vi "Format Memory Cell to String.vi"(8 "error in (no error)":errorcluster, 10 "Format String":string, 11 "Memory Cell":T1) -> (0 "error out":errorcluster, 3 "output string":string)   [LabVIEW 2024]
uses:
  gScript Interpreter/Type Definitions/Memory Cell.ctl
  gScript Interpreter/Type Definitions/Memory Cell Type Enum.ctl
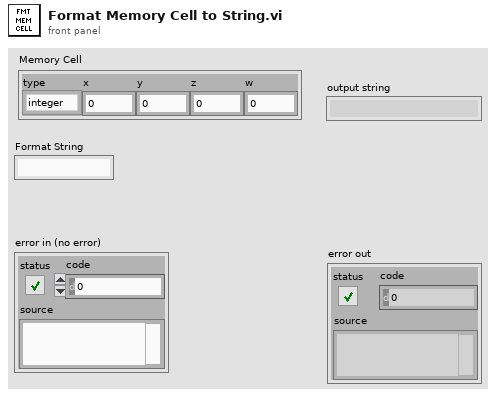
[diagram p1: front panel]
types:
  T1 = typedef "Memory Cell.ctl" = cluster{"type":T2, "x":dbl, "y":dbl, "z":dbl, "w":dbl}
  T2 = typedef "Memory Cell Type Enum.ctl" = enum16{"integer", "float", "vector", "rotation"}
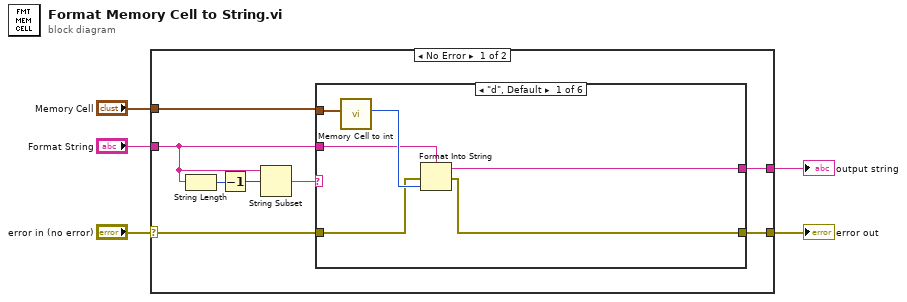
[diagram p0: block diagram]
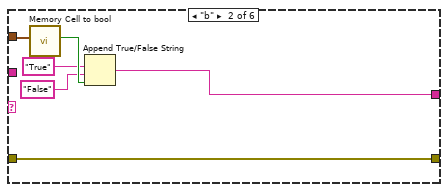
[diagram p2: hidden frame]
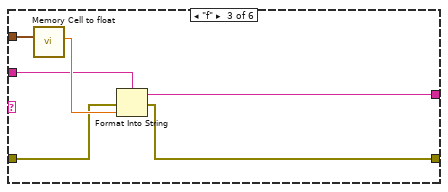
[diagram p3: hidden frame]
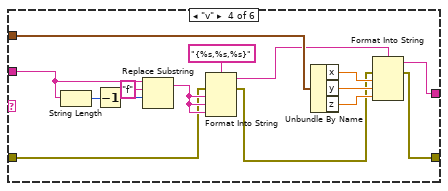
[diagram p4: hidden frame]
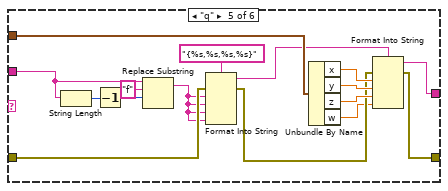
[diagram p5: hidden frame]
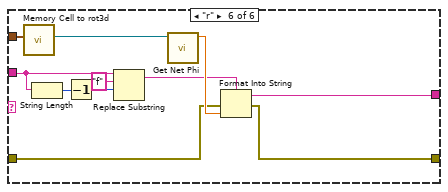
[diagram p6: hidden frame]
diagram:
  n1 = case shown="No Error" "error in (no error)" {
    selector: "error in (no error)" -> [w8 w74]
    tunnel: [w7 w74] -> w4
    tunnel: "Format String" -> [w9 _]
    tunnel: "Memory Cell" -> [w11 _]
    tunnel: [w6 _] -> w1
    frame No Error {
      n2 = String Length(string=w9) -> (length=w13:i32)
      n3 = Decrement(x=w13) -> (x-1=w12:i32)
      n4 = String Subset(string=w9, offset (0)=w12) -> (substring=w10:string)  [unwired: 1 in]
      n5 = case shown="\"d\", Default" w10 {
        tunnel: w11 -> [w19 w25 w31 w46 w62 w73]
        tunnel: [w14 w21 w29 w32 w48 w63] -> w6
        tunnel: w9 -> [w17 _ w26 w41 w57 w67]
        tunnel: w8 -> [w16 w20 w28 w36 w53 w65]
        tunnel: [w15 w20 w27 w34 w51 w64] -> w7
        frame "d", Default {
          n6 = call "Memory Cell to int.vi"("Memory Cell"=w19) -> ("Int out"=w18:i32)  [unwired: 10 in]
          n7 = Format Into String(format string=w17, error in=w16, w18) -> (resulting string=w14:string, error out=w15:errorcluster)  [unwired: 1 in]
        }
        frame "b" {
          n8 = call "Memory Cell to bool.vi"("Memory Cell"=w25) -> ("bool out"=w24:bool)  [unwired: 10 in]
          n9 = Append True/False String(1:w24, 2:"False" ("false string"), 3:"True" ("true string")) -> (0:w21:string)  [unwired: 1 in]
        }
        frame "f" {
          n10 = call "Memory Cell to float.vi"("Memory Cell"=w31) -> ("float out"=w30:dbl)  [unwired: 10 in]
          n11 = Format Into String(format string=w26, error in=w28, w30) -> (resulting string=w29:string, error out=w27:errorcluster)  [unwired: 1 in]
        }
        frame "v" {
          n12 = String Length(string=w41) -> (length=w42:i32)
          n13 = Decrement(x=w42) -> (x-1=w40:i32)
          n14 = Replace Substring(3:w40, 4:"f" ("substring (\"\")"), 5:w41) -> (1:w37:string)  [unwired: 1 in, 1 out]
          n15 = Format Into String(format string="{%s,%s,%s}", error in=w36, w37, w37, w37) -> (resulting string=w33:string, error out=w35:errorcluster)  [unwired: 1 in]
          n16 = Unbundle By Name(w46) -> ("x"=w45:dbl, "y"=w44:dbl, "z"=w43:dbl)
          n17 = Format Into String(format string=w33, error in=w35, w45, w44, w43) -> (resulting string=w32:string, error out=w34:errorcluster)  [unwired: 1 in]
        }
        frame "q" {
          n18 = String Length(string=w57) -> (length=w58:i32)
          n19 = Decrement(x=w58) -> (x-1=w56:i32)
          n20 = Replace Substring(3:w56, 4:"f" ("substring (\"\")"), 5:w57) -> (1:w49:string)  [unwired: 1 in, 1 out]
          n21 = Format Into String(format string="{%s,%s,%s,%s}", error in=w53, w49, w49, w49, w49) -> (resulting string=w50:string, error out=w52:errorcluster)  [unwired: 1 in]
          n22 = Unbundle By Name(w62) -> ("x"=w61:dbl, "y"=w60:dbl, "z"=w59:dbl, "w"=w47:dbl)
          n23 = Format Into String(format string=w50, error in=w52, w61, w60, w59, w47) -> (resulting string=w48:string, error out=w51:errorcluster)  [unwired: 1 in]
        }
        frame "r" {
          n24 = call "Memory Cell to rot3d.vi"("Memory Cell"=w73) -> ("Orient3d out"=w72:refnum<class "Orient3d.lvclass">)  [unwired: 10 in]
          n25 = String Length(string=w67) -> (length=w70:i32)
          n26 = Decrement(x=w70) -> (x-1=w69:i32)
          n27 = Replace Substring(3:w69, 4:"f" ("substring (\"\")"), 5:w67) -> (1:w66:string)  [unwired: 1 in, 1 out]
          n28 = call "Get Net Phi.vi"("Orient3d"=w72) -> ("phi(deg)"=w71:dbl)  [unwired: 8 in, 2 out]
          n29 = Format Into String(format string=w66, error in=w65, w71) -> (resulting string=w63:string, error out=w64:errorcluster)  [unwired: 1 in]
        }
      }
    }
    frame Error {
    }
  }
  "error out" <- w4
  "output string" <- w1
